vi "fg_file.vi"(8 "error in (no error)":errorcluster, 11 "files":T1) -> (0 "error out":errorcluster, 3 "file":path)   [LabVIEW 2015, in "lv-bin-7zip.lvlib"]
uses:
  lv-bin-7zip.lvlib
  _controls/files.ctl
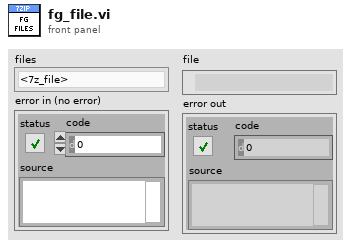
[diagram p1: front panel]
types:
  T1 = typedef "lv-bin-7zip.lvlib/files.ctl" = enum16{"<7z_file>", "7z.dll", "7z.exe", "7z.sfx", "7zCon.sfx", "7zFM. exe", "7zG.exe"}
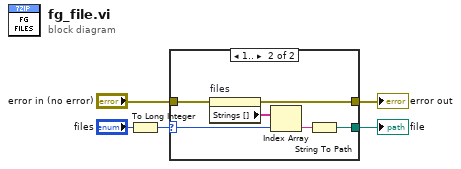
[diagram p0: block diagram]
diagram:
  n1 = To Long Integer(number="files") -> (32bit integer=w1:i32)
  n2 = case shown="1.." w1 {
    selector: w1 -> [_ w7]
    tunnel: "error in (no error)" -> [w6 w12]
    tunnel: [w6 w11] -> w4
    tunnel: [_ w8] -> w2
    frame Default {
    }
    frame 1.. {
      n3 = property on="files" class="Enum (strict)"(error in=w12) -> (error out=w11:errorcluster, "Strings []"=w10:string[])  [unwired: 1 in, 1 out]
      n4 = Index Array(array=w10, index=w7) -> (element=w9:string)
      n5 = String To Path(string=w9) -> (path=w8:path)
    }
  }
  "error out" <- w4
  "file" <- w2
